vi "Initialize.vi"(8 "error in":errorcluster, 10 "sPanel":refnum<vi>, 11 "GUI Facade in":refnum<class "GUI Facade.lvclass">) -> (0 "error out":errorcluster, 3 "GUI Facade out":refnum<class "GUI Facade.lvclass">)   [LabVIEW 2018, in "GUI Facade.lvclass"]
doc: "The initialize function is abstract as the layout will be dependent on the implementation."
uses:
  GUI Facade.lvclass
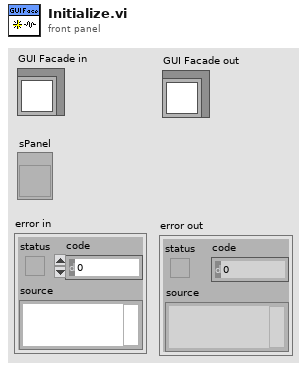
[diagram p1: front panel]
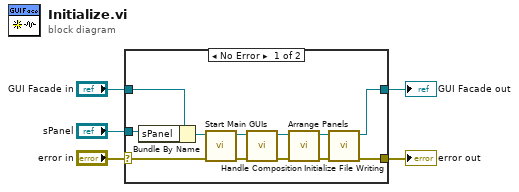
[diagram p0: block diagram]
diagram:
  n1 = case shown="No Error" "error in" {
    selector: "error in" -> [w10 w19]
    tunnel: [w7 w19] -> w4
    tunnel: [w6 w18] -> w2
    tunnel: "GUI Facade in" -> [w17 w18]
    tunnel: "sPanel" -> [w16 _]
    frame No Error {
      n2 = Bundle By Name(cluster=w17, "sPanel"=w16) -> (w15:refnum<class "GUI Facade.lvclass">)
      n3 = call-dynamic "Start Main GUIs.vi"("error in (no error)"=w10, "GUI Facade in"=w15) -> ("error out"=w13:errorcluster, "GUI Facade out"=w14:refnum<class "GUI Facade.lvclass">)  [unwired: 8 in]
      n4 = call-dynamic "Handle Composition.vi"("error in (no error)"=w13, "GUI Facade in"=w14) -> ("error out"=w11:errorcluster, "GUI Facade out"=w12:refnum<class "GUI Facade.lvclass">)  [unwired: 8 in]
      n5 = call-dynamic "Arrange Panels.vi"("error in (no error)"=w11, "GUI Facade in"=w12) -> ("error out"=w8:errorcluster, "GUI Facade out"=w9:refnum<class "GUI Facade.lvclass">)  [unwired: 8 in]
      n6 = call-dynamic "Initialize File Writing.vi"("error in"=w8, "GUI Facade in"=w9) -> ("error out"=w7:errorcluster, "GUI Facade out"=w6:refnum<class "GUI Facade.lvclass">)  [unwired: 8 in]
    }
    frame Error {
    }
  }
  "error out" <- w4
  "GUI Facade out" <- w2
